vi "Mark beam Locations.vi"(10 "Track Point":T1[](array[typedef]), 11 "Array in":bool[][](array[boolean])) -> (3 "Array in 2":bool[][](array[boolean]))   [LabVIEW 2023]
uses:
  Cluster_Tracking point.ctl
  Cluster_Point.ctl
  ENUM_Direction_a2.ctl
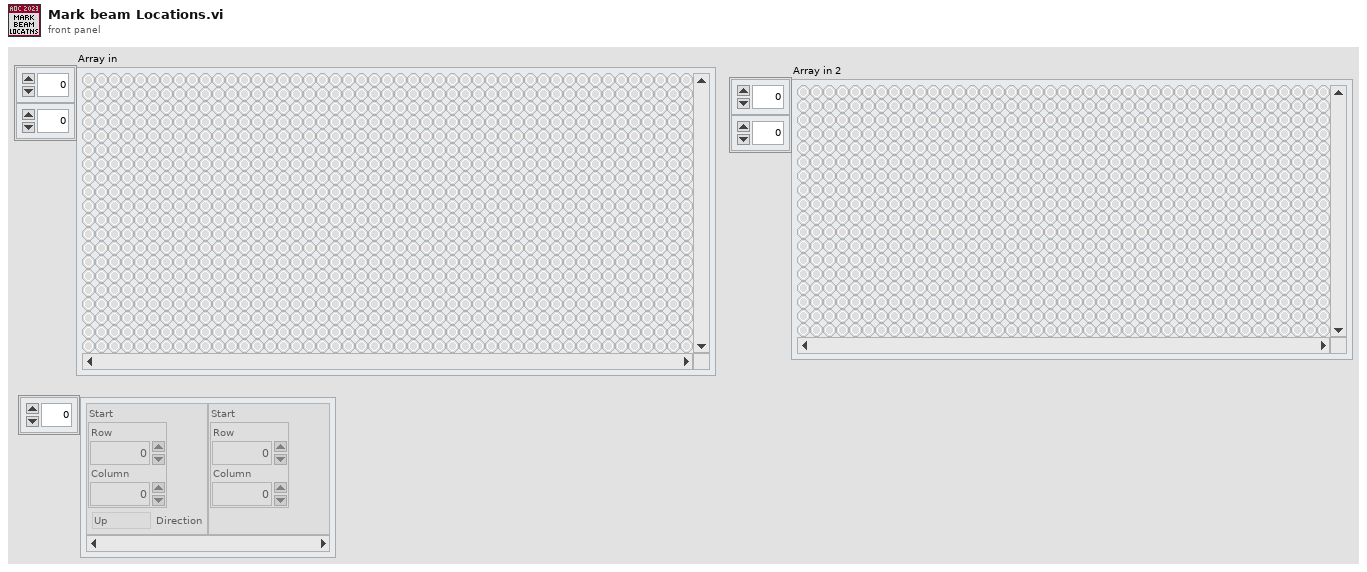
[diagram p1: front panel]
types:
  T1 = typedef "Cluster_Tracking point.ctl" = cluster{"Start":T2, "Direction":T3}
  T2 = typedef "Cluster_Point.ctl" = cluster{"Row":i32, "Column":i32}
  T3 = typedef "ENUM_Direction_a2.ctl" = enum16{"Up", "Left", "Down", "Right", "Up-Down", "Left-Right"}
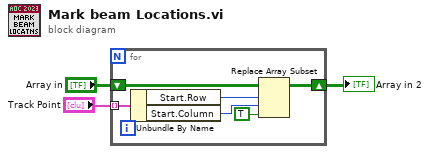
[diagram p0: block diagram]
diagram:
  n1 = for {
    shift-right: [w7] -> w2
    shift-left: "Array in" -> [w8]
    tunnel: "Track Point" -> [w9] mode=indexing
    n2 = Unbundle By Name(w9) -> ("Start.Row"=w6:i32, "Start.Column"=w5:i32)
    n3 = Replace Array Subset(array=w8, new element=TRUE ("new element/subarray"), index (row)=w6, index (col)=w5) -> (w7:bool[][])
  }
  "Array in 2" <- w2
